vi "获取网络连接状态.vi"() -> (0 "网络连接状态":bool)   [LabVIEW 2015]
uses:
  wininet.dll
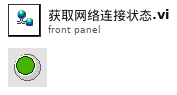
[diagram p1: front panel]
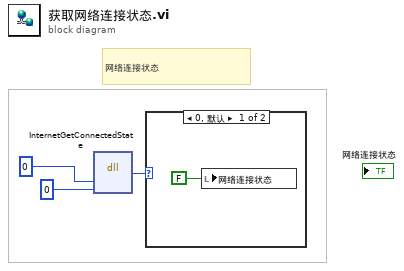
[diagram p0: block diagram]
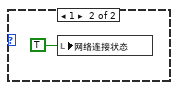
[diagram p2: hidden frame]
diagram:
  # "网络连接状态"
  n1 = dll-call lib="wininet.dll" fn="InternetGetConnectedState"("one"=u32 0, "two"=u32 0) -> ("返回类型"=w1:u32)  [unwired: 5 in, 2 out]
  n2 = case shown="0, 默认" w1 {
    frame 0, Default {
      n3 = local write "网络连接状态"(FALSE ("断网提醒")) -> ()
    }
    frame 1 {
      n4 = local write "网络连接状态"(TRUE ("断网提醒")) -> ()
    }
  }
